vi "Parallax PING Read Distance.vi"(8 "error in (no error)":errorcluster, 10 "Temperature (deg C)":dbl=30.0, 11 "myRIO DIO Channel":tag="C/DIO1") -> (0 "error out":errorcluster, 3 "Distance (m)":dbl)   [LabVIEW 2019]
doc: "Reads the distance in meters from the Parallax PING sensor located on the given pin.\n\nReturns -1 if the distance could not be read."
uses:
  <vilib>/myRIO/Instrument Drivers/Onboard IO/DIO/typedefs/DIO Reference.ctl
  <vilib>/myRIO/Common/Instrument Driver Framework/Utilities/typedefs/myRIO Generic Hardware Reference.ctl
  <vilib>/myRIO/Common/Instrument Driver Framework/Utilities/typedefs/Hardware Version Enum.ctl
  <vilib>/myRIO/Common/Instrument Driver Framework/Utilities/typedefs/myRIO v1.0 Reference.ctl
  <vilib>/myRIO/Common/Instrument Driver Framework/Utilities/typedefs/Generic FPGA Reference.ctl
  <vilib>/myRIO/Common/Instrument Driver Framework/myRIO v1.0/DIO/typedefs/DIO Channels List.ctl
  <vilib>/myRIO/Common/Instrument Driver Framework/myRIO v1.0/DIO/typedefs/DIO Channels Enum.ctl
  <vilib>/myRIO/Common/Instrument Driver Framework/myRIO v1.0/DIO/vis/myRIO v1.0 Close DIO.vi
  <vilib>/myRIO/Common/Instrument Driver Framework/myRIO v1.0/DIO/vis/myRIO v1.0 Unreserve DIO.vi
  <vilib>/myRIO/Common/Instrument Driver Framework/myRIO v1.0/DIO/vis/myRIO v1.0 Build MUX Configuration DIO.vi
  <vilib>/myRIO/Common/Instrument Driver Framework/myRIO v1.0/Resource Manager/vis/myRIO v1.0 Unreserve Channel List.vi
  <vilib>/myRIO/Common/Instrument Driver Framework/myRIO v1.0/Resource Manager/vis/myRIO v1.0 Create Configuration List.vi
  <vilib>/myRIO/Common/Instrument Driver Framework/myRIO v1.0/Resource Manager/vis/myRIO v1.0 Unreserve Channel.vi
  <vilib>/myRIO/Common/Instrument Driver Framework/myRIO v1.0/Resource Manager/vis/myRIO v1.0 Build Mutex Name.vi
  <vilib>/Utility/error.llb/Error Cluster From Error Code.vi
  <vilib>/myRIO/Common/Instrument Driver Framework/myRIO v1.0/DIO/vis/myRIO v1.0 Write DIO.vi
  <vilib>/myRIO/Common/Instrument Driver Framework/myRIO v1.0/DIO/vis/myRIO v1.0 Read DIO.vi
  <vilib>/myRIO/Common/Instrument Driver Framework/myRIO v1.0/DIO/vis/myRIO v1.0 Shutdown DIO.vi
  <vilib>/myRIO/Common/Instrument Driver Framework/myRIO v1.0/Resource Manager/vis/myRIO v1.0 Configure IO.vi
  <vilib>/myRIO/Common/Instrument Driver Framework/Utilities/vis/Configuration Manager.vi
  <vilib>/myRIO/Common/Instrument Driver Framework/Utilities/vis/IO Manager.vi
  <vilib>/myRIO/Common/Instrument Driver Framework/myRIO v1.0/myRIO v1.0 Close.vi
  <vilib>/myRIO/Instrument Drivers/Onboard IO/DIO/DIO.lvlib
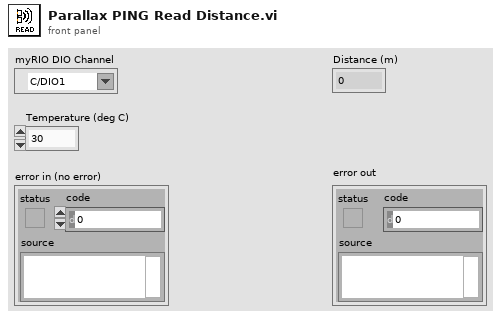
[diagram p1: front panel]
types:
  T1 = enum16{"Initialize", "Trigger pulse", "Wait for rising edge", "Wait for falling edge", "Calculate distance", "Stop"}
  T2 = typedef "DIO.lvlib/DIO Reference.ctl" = cluster{"myRIO Reference":T3, "DIO Channels List":T7}
  T3 = typedef "myRIO Generic Hardware Reference.ctl" = cluster{"myRIO Model":T4, "myRIO Hardware Reference":T5}
  T4 = typedef "Hardware Version Enum.ctl" = enum16{"Unknown", "myRIO-1900", "myRIO-1950", "roboRIO", "NI ELVIS RIO CM", "ELVIS III"}
  T5 = typedef "myRIO v1.0 Reference.ctl" = cluster{"Generic FPGA Reference":T6, "Allow multiple opens":bool}
  T6 = typedef "Generic FPGA Reference.ctl" = refnum<k20>
  T7 = typedef "DIO Channels List.ctl" = T8[]
  T8 = typedef "DIO Channels Enum.ctl" = enum16{"Not Connected", "C/DIO0", "C/DIO1", "C/DIO2", "C/DIO3", "C/DIO4", "C/DIO5", "C/DIO6", "C/DIO7", "A/DIO0", "A/DIO1", "A/DIO2", "A/DIO3", "A/DIO4", "A/DIO5", "A/DIO6", "A/DIO7", "A/DIO8", "A/DIO9", "A/DIO10", "A/DIO11", "A/DIO12", "A/DIO13", "A/DIO14", "A/DIO15", "A/DIO16", "A/DIO17", "A/DIO18", "A/DIO19", "B/DIO0", "B/DIO1", "B/DIO2", "B/DIO3", "B/DIO4", "B/DIO5", "B/DIO6", "B/DIO7", "B/DIO8", "B/DIO9", "B/DIO10", "B/DIO11", "B/DIO12", "B/DIO13", "B/DIO14", "B/DIO15", "B/DIO16", "B/DIO17", "B/DIO18", "B/DIO19", "LED0", "LED1", "LED2", "LED3", "Button0", "DIO/DIO0", "DIO/DIO1", "DIO/DIO2", "DIO/DIO3", "DIO/DIO4", "DIO/DIO5", "DIO/DIO6", "DIO/DIO7", "DIO/DIO8", "DIO/DIO9", "SPI/CS0", "SPI/CS1", "SPI/CS2", "SPI/CS3", "LED RADIO (Green)", "LED RADIO (Red)", "LED COMM (Green)", "LED COMM (Red)", "LED MODE (Green)", "LED MODE (Red)"}
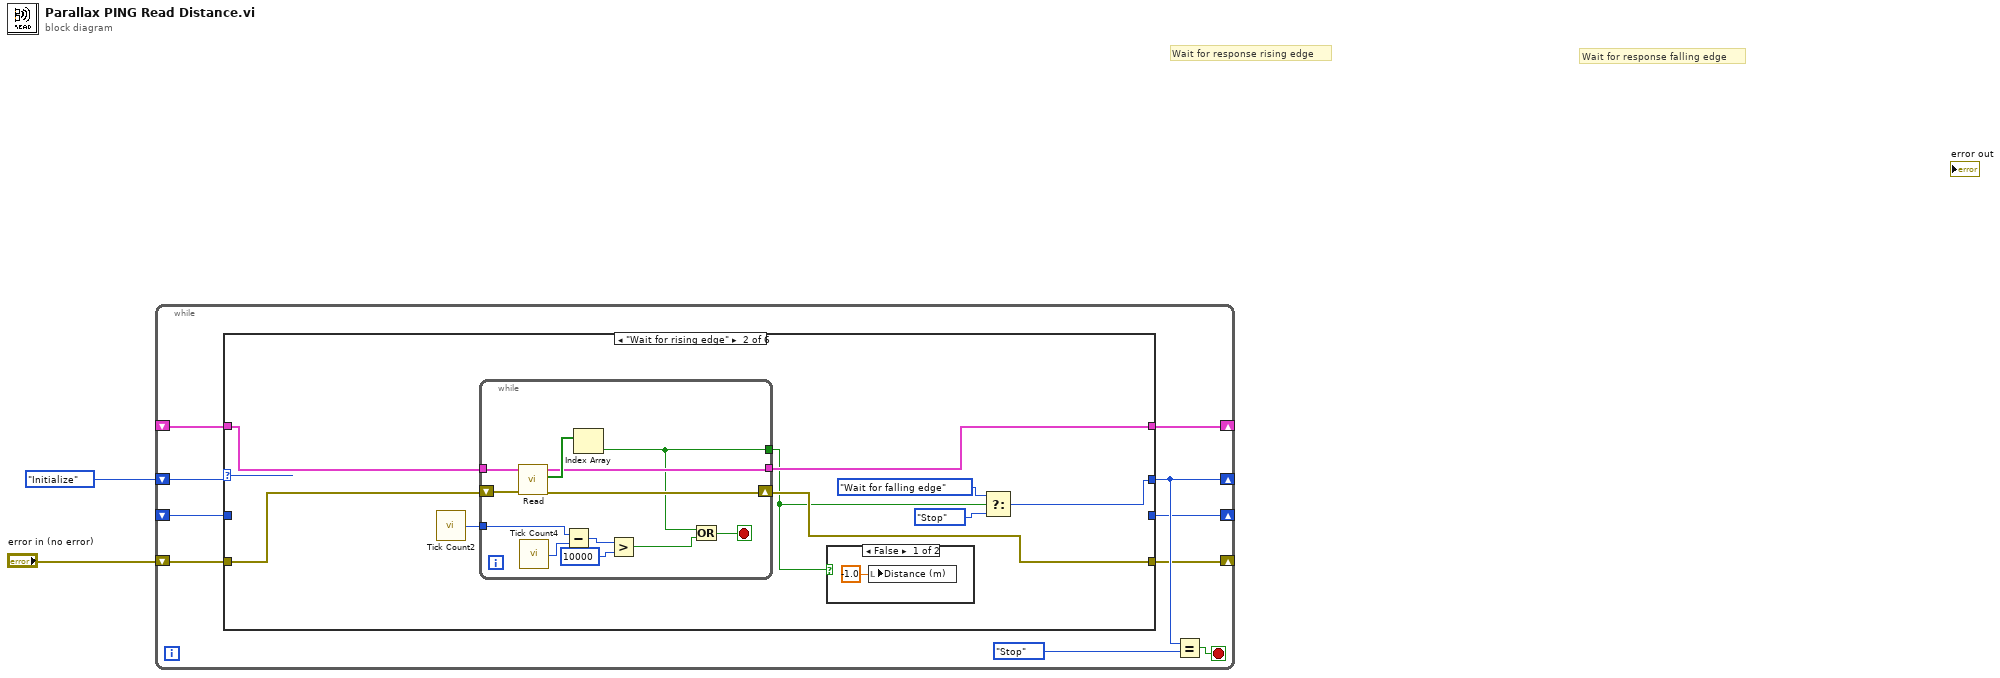
[diagram p0: block diagram]
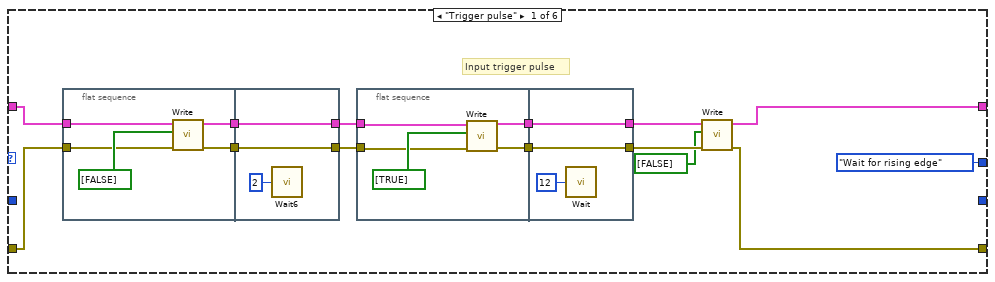
[diagram p2: hidden frame]
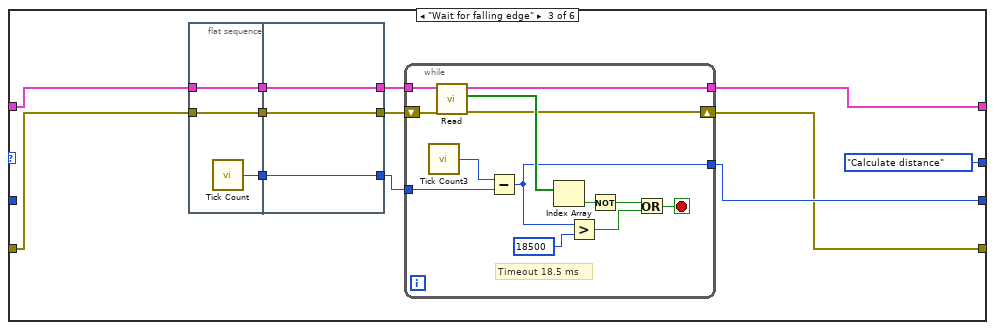
[diagram p4: hidden frame]
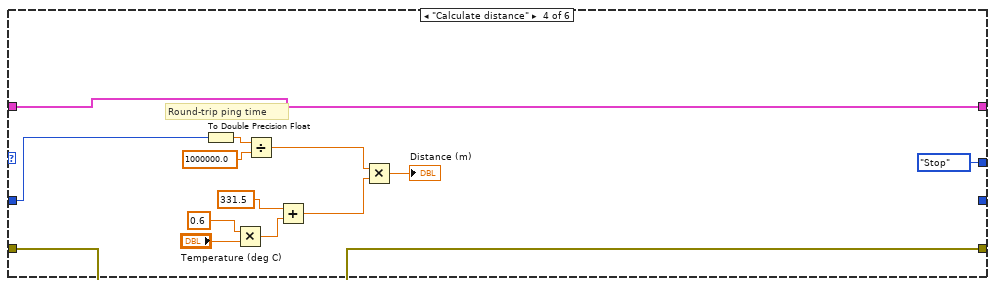
[diagram p5: hidden frame]
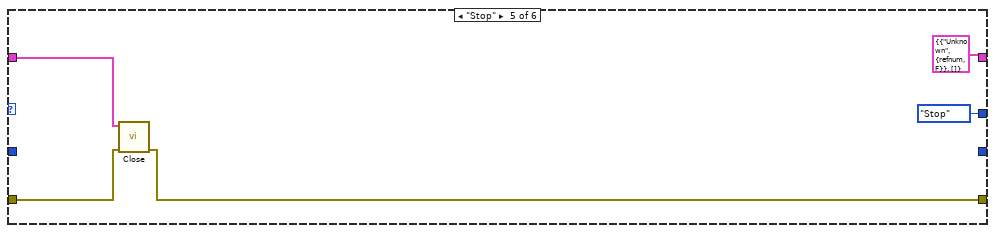
[diagram p6: hidden frame]
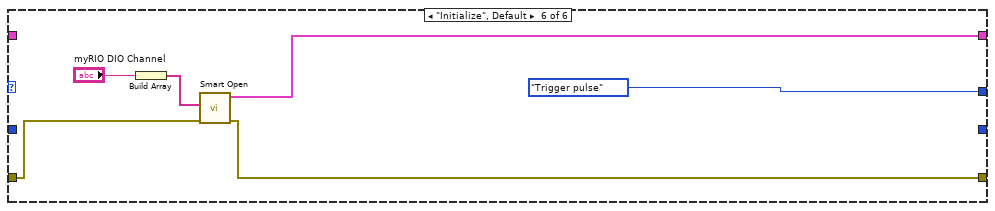
[diagram p7: hidden frame]
diagram:
  # "Wait for response falling edge"
  # "Wait for response rising edge"
  n1 = while {
    shift-right: [w11] -> _
    shift-left: T1."Initialize" -> [w10]
    shift-right: [w5] -> _
    shift-left: "error in (no error)" -> [w8]
    shift-right: [w7] -> _
    shift-left: _ -> [w6]
    shift-right: [w4] -> _
    shift-left: _ -> [w3]
    stop <- w12 stop-if-true
    n2 = case shown="\"Wait for rising edge\"" w10 {
      tunnel: [T1."Wait for rising edge" w49 T1."Calculate distance" ("y") T1."Stop" ("y") T1."Stop" ("y") T1."Trigger pulse"] -> w11
      tunnel: w8 -> [w17 w43 w69 w96 w112 w117]
      tunnel: [w15 w48 w68 w99 T2 {"myRIO Reference"={"myRIO Model"=enum."Unknown", "myRIO Hardware Reference"={"Generic FPGA Reference"=refnum, "Allow multiple opens"=FALSE}}, "DIO Channels List"=[]} ("DIO Ref Out") w116] -> w7
      tunnel: w6 -> [w16 w44 w70 w99 w111 _]
      tunnel: [w14 w47 w65 w96 w110 w115] -> w5
      tunnel: [_ _ w67 _ _ _] -> w4
      tunnel: w3 -> [_ _ _ w98 _ _]
      frame "Trigger pulse" {
        # "Input trigger pulse"
        n3 = flat-sequence {
          tunnel: [w30] -> w24
          tunnel: [w29] -> w23
          tunnel: w17 -> [w28]
          tunnel: w16 -> [w27]
          tunnel: [w33] -> w21
          tunnel: [w32] -> w22
          tunnel: w24 -> [w33]
          tunnel: w23 -> [w32]
          frame #0 {
            n4 = call <vilib>:"Write.vi"("error in (no error)"=w28, "Values"=bool[] [FALSE], "DIO Ref In"=w27) -> ("error out"=w29:errorcluster, "DIO Ref Out"=w30:T2)  [unwired: 6 in]
          }
          frame #1 {
            n5 = call "Wait6"("Count(uSec)"=u32 2) -> ()  [unwired: 1 out]
          }
        }
        n6 = flat-sequence {
          tunnel: [w38] -> w26
          tunnel: [w37] -> w25
          tunnel: w22 -> [w36]
          tunnel: w21 -> [w35]
          tunnel: [w41] -> w18
          tunnel: [w40] -> w20
          tunnel: w26 -> [w41]
          tunnel: w25 -> [w40]
          frame #0 {
            n7 = call <vilib>:"Write.vi"("error in (no error)"=w36, "Values"=bool[] [TRUE], "DIO Ref In"=w35) -> ("error out"=w37:errorcluster, "DIO Ref Out"=w38:T2)  [unwired: 6 in]
          }
          frame #1 {
            n8 = call "Wait"("Count(uSec)"=u32 12) -> ()  [unwired: 1 out]
          }
        }
        n9 = call <vilib>:"Write.vi"("error in (no error)"=w20, "Values"=bool[] [FALSE], "DIO Ref In"=w18) -> ("error out"=w14:errorcluster, "DIO Ref Out"=w15:T2)  [unwired: 6 in]
      }
      frame "Wait for rising edge" {
        n10 = call "Tick Count2"() -> ("Tick Count(uSec)"=w45:u32)
        n11 = while {
          tunnel: [w63] -> w48
          shift-right: [w61] -> w47
          shift-left: w43 -> [w62]
          tunnel: w45 -> [w58]
          tunnel: w44 -> [w60]
          tunnel: [w53] -> w46
          stop <- w55 stop-if-true
          n12 = call <vilib>:"Read.vi"("error in (no error)"=w62, "DIO Ref In"=w60) -> ("error out"=w61:errorcluster, "Values"=w64:bool[], "DIO Ref Out"=w63:T2)  [unwired: 7 in]
          n13 = call "Tick Count4"() -> ("Tick Count(uSec)"=w59:u32)
          n14 = Subtract(x=w58, y=w59) -> (x-y=w57:u32)
          n15 = Index Array(array=w64) -> (element=w53:bool)  [unwired: 1 in]
          n16 = Greater?(x=w57, y=u32 10000) -> (0:w54:bool)
          n17 = Or(x=w53, y=w54) -> (x .or. y?=w55:bool)
        }
        n18 = case shown="False" w46 {
          frame False {
            n19 = local write "Distance (m)"(-1.0 ("Distance (m)")) -> ()
          }
          frame True {
          }
        }
        n20 = Select(t=T1."Wait for falling edge", s=w46, f=T1."Stop" ("y")) -> (s? t:f=w49:T1)
      }
      frame "Wait for falling edge" {
        n21 = flat-sequence {
          tunnel: w70 -> [w92]
          tunnel: [w92] -> w76
          tunnel: [w91] -> w75
          tunnel: [w90] -> w74
          tunnel: w69 -> [w90]
          tunnel: [w94] -> w72
          tunnel: [w95] -> w73
          tunnel: w76 -> [w95]
          tunnel: w75 -> [w94]
          tunnel: w74 -> [w93]
          tunnel: [w93] -> w71
          frame #0 {
            n22 = call "Tick Count"() -> ("Tick Count(uSec)"=w91:u32)
          }
          frame #1 {
          }
        }
        n23 = while {
          tunnel: w73 -> [w89]
          tunnel: w72 -> [w86]
          shift-right: [w80] -> w65
          shift-left: w71 -> [w81]
          tunnel: [w78] -> w68
          tunnel: [w77] -> w67
          stop <- w85 stop-if-true
          # "Timeout 18.5 ms"
          n24 = call "Tick Count3"() -> ("Tick Count(uSec)"=w79:u32)
          n25 = call <vilib>:"Read.vi"("error in (no error)"=w81, "DIO Ref In"=w89) -> ("error out"=w80:errorcluster, "Values"=w88:bool[], "DIO Ref Out"=w78:T2)  [unwired: 7 in]
          n26 = Subtract(x=w79, y=w86) -> (x-y=w77:u32)
          n27 = Index Array(array=w88) -> (element=w87:bool)  [unwired: 1 in]
          n28 = Greater?(x=w77, y=u32 18500) -> (0:w83:bool)
          n29 = Not(x=w87) -> (.not. x?=w84:bool)
          n30 = Or(x=w84, y=w83) -> (x .or. y?=w85:bool)
        }
      }
      frame "Calculate distance" {
        # "Round-trip ping time"
        n31 = To Double Precision Float(number=w98) -> (double precision float=w104:dbl)
        n32 = Multiply(x=0.6, y="Temperature (deg C)") -> (x*y=w102:dbl)
        n33 = Divide(x=w104, y=1000000.0) -> (x/y=w106:dbl)
        n34 = Add(x=331.5, y=w102) -> (x+y=w107:dbl)
        n35 = Multiply(x=w106, y=w107) -> (x*y=→"Distance (m)":dbl)
      }
      frame "Stop" {
        n36 = call <vilib>:"Close.vi"("error in (no error)"=w112, "DIO Ref In"=w111) -> ("error out"=w110:errorcluster)  [unwired: 9 in]
      }
      frame "Initialize", Default {
        n37 = Build Array("myRIO DIO Channel") -> (w119:tag[])
        n38 = call <vilib>:"Smart Open.vi"("error in (no error)"=w117, "Channel Names"=w119) -> ("error out"=w115:errorcluster, "DIO Ref Out"=w116:T2)  [unwired: 8 in]
      }
    }
    n39 = Equal?(x=w11, y=T1."Stop") -> (x = y?=w12:bool)
  }
